vi "List Project Build Specifications.vi"(8 "error in (no error)":errorcluster, 10 "project path":path) -> (0 "error out":errorcluster, 3 "Build Specs":T1[](array[typedef]))   [LabVIEW 2019, in "ProjectItem.lvclass"]
uses:
  Build/Typedefs/Build Spec--cluster.ctl
  <vilib>/xml/Load XML File.vi
  <vilib>/xml/Close Reference(Node).vi
  ProjectItem.lvclass
  <vilib>/xml/NI_XML.lvlib
  Build/Build.lvlib
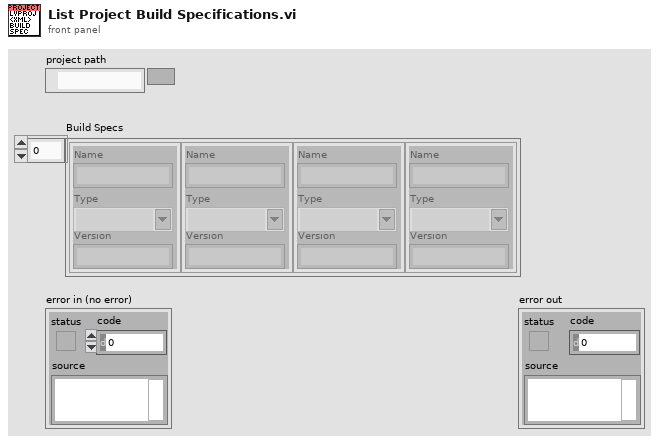
[diagram p1: front panel]
types:
  T1 = typedef "Build.lvlib/Build Spec--cluster.ctl" = cluster{"Name":string, "Type":string, "Version":string}
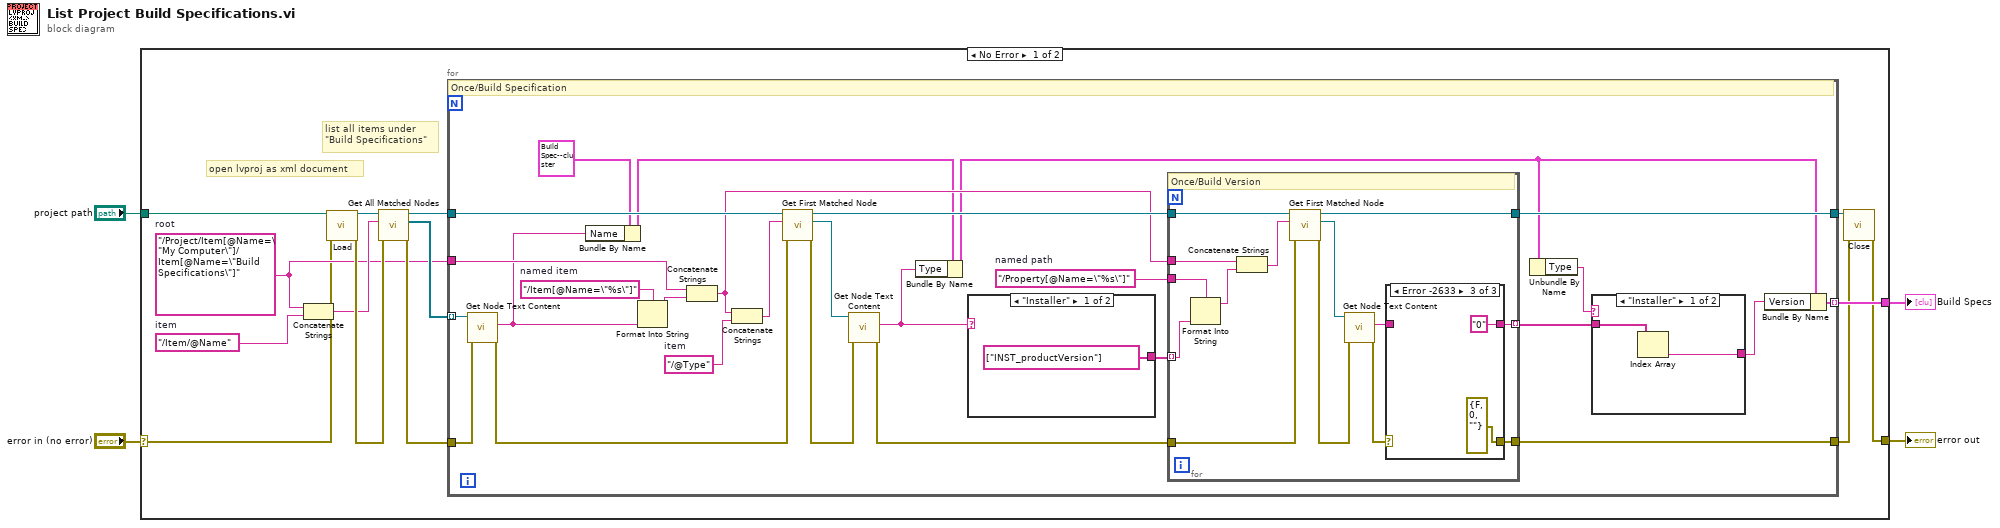
[diagram p0: block diagram]
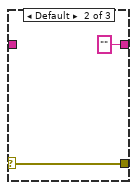
[diagram p3: hidden frame]
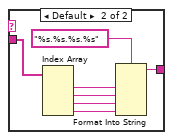
[diagram p4: hidden frame]
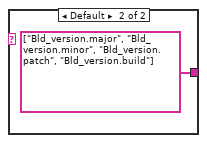
[diagram p5: hidden frame]
diagram:
  n1 = case shown="No Error" "error in (no error)" {
    selector: "error in (no error)" -> [w7 w77]
    tunnel: "project path" -> [w18 _]
    tunnel: [w17 _] -> w3
    tunnel: [w6 w77] -> w1
    frame No Error {
      w5 = "/Item/@Name"  # item
      w10 = "/Project/Item[@Name=\"My Computer\"]/Item[@Name=\"Build Specifications\"]"  # root
      # "list all items under\n\"Build Specifications\""
      # "open lvproj as xml document"
      n2 = Concatenate Strings(w10, w5) -> (w11:string)
      n3 = call-poly <vilib>:"Load.vi"("path to XML document"=w18, "error in (no error)"=w7) -> ("DOM document out"=w16:refnum<k20>, "error out"=w15:errorcluster)  [unwired: 11 in, 1 out]
      n4 = call <vilib>:"Get All Matched Nodes.vi"("error in (no error)"=w15, "XPath expression"=w11, "node in"=w16) -> ("error out"=w12:errorcluster, "node result array"=w14:refnum<k20>[], "node out"=w13:refnum<k20>)  [unwired: 6 in]
      n5 = for {
        tunnel: w14 -> [w45] mode=indexing
        tunnel: w13 -> [w44]
        tunnel: w10 -> [w25]
        tunnel: w12 -> [w43]
        tunnel: [w29] -> w9
        tunnel: [w26] -> w17 mode=indexing
        tunnel: [w31] -> w8
        w35 = "/Property[@Name=\"%s\"]"  # named path
        w37 = "/@Type"  # item
        w39 = "/Item[@Name=\"%s\"]"  # named item
        # "Once/Build Specification"
        n6 = call <vilib>:"Get Node Text Content.vi"("error in (no error)"=w43, "node in"=w45) -> ("error out"=w42:errorcluster, "node text"=w21:string)  [unwired: 7 in, 1 out]
        n7 = Bundle By Name(cluster=T1 {"Name"="My Application", "Type"="EXE", "Version"="1.0.0.1"} ("BuildSpec"), "Name"=w21) -> (w20:T1)
        n8 = Format Into String(format string=w39, w21) -> (resulting string=w38:string)  [unwired: 2 in, 1 out]
        n9 = Concatenate Strings(w25, w38) -> (w30:string)
        n10 = Concatenate Strings(w30, w37) -> (w36:string)
        n11 = call <vilib>:"Get First Matched Node.vi"("error in (no error)"=w42, "XPath expression"=w36, "node in"=w44) -> ("error out"=w40:errorcluster, "node result"=w41:refnum<k20>, "node out"=w33:refnum<k20>)  [unwired: 6 in]
        n12 = call <vilib>:"Get Node Text Content.vi"("error in (no error)"=w40, "node in"=w41) -> ("error out"=w32:errorcluster, "node text"=w23:string)  [unwired: 7 in, 1 out]
        n13 = Bundle By Name(cluster=w20, "Type"=w23) -> (w24:T1)
        n14 = case shown="\"Installer\"" w23 {
          tunnel: [string[] ["INST_productVersion"] ("XPath expression") string[] ["Bld_version.major", "Bld_version.minor", "Bld_version.patch", "Bld_version.build"] ("XPath expression")] -> w34
          frame "Installer" {
          }
          frame Default {
          }
        }
        n15 = for {
          tunnel: w35 -> [w59]
          tunnel: w34 -> [w58] mode=indexing
          tunnel: w33 -> [w53]
          tunnel: w32 -> [w52]
          tunnel: [w46] -> w31
          tunnel: w30 -> [w51]
          tunnel: [w50] -> w29
          tunnel: [w48] -> w28 mode=indexing
          # "Once/Build Version"
          n16 = Format Into String(format string=w59, w58) -> (resulting string=w56:string)  [unwired: 2 in, 1 out]
          n17 = Concatenate Strings(w51, w56) -> (w55:string)
          n18 = call <vilib>:"Get First Matched Node.vi"("error in (no error)"=w52, "XPath expression"=w55, "node in"=w53) -> ("error out"=w54:errorcluster, "node result"=w57:refnum<k20>, "node out"=w50:refnum<k20>)  [unwired: 6 in]
          n19 = call <vilib>:"Get Node Text Content.vi"("error in (no error)"=w54, "node in"=w57) -> ("error out"=w49:errorcluster, "node text"=w47:string)  [unwired: 7 in, 1 out]
          n20 = case shown="Error -2633" w49 {
            selector: w49 -> [w60 w63 _]
            tunnel: [w61 "" ("node text") "0" ("node text")] -> w48
            tunnel: w47 -> [w61 _ _]
            tunnel: [w60 w63 errorcluster {"status"=FALSE, "code"=0, "source"=""} ("error IO")] -> w46
            frame No Error {
            }
            frame Default {
            }
            frame Error {
            }
          }
        }
        n21 = Unbundle By Name(w24) -> ("Type"=w22:string)
        n22 = case shown="\"Installer\"" w22 {
          tunnel: w28 -> [w67 w73]
          tunnel: [w66 w68] -> w27
          frame "Installer" {
            n23 = Index Array(array=w67) -> (element=w66:string)  [unwired: 1 in]
          }
          frame Default {
            n24 = Index Array(array=w73) -> (element #1=w72:string, element #2=w69:string, element #3=w70:string, element #4=w71:string)  [unwired: 4 in]
            n25 = Format Into String(format string="%s.%s.%s.%s", w72, w69, w70, w71) -> (resulting string=w68:string)  [unwired: 2 in, 1 out]
          }
        }
        n26 = Bundle By Name(cluster=w24, "Version"=w27) -> (w26:T1)
      }
      n27 = call-poly <vilib>:"Close.vi"("error in (no error)"=w8, "node"=w9) -> ("error out"=w6:errorcluster)  [unwired: 7 in]
    }
    frame Error {
    }
  }
  "Build Specs" <- w3
  "error out" <- w1
